vi "Format 2D Test Info Table.vi"(1 "Parameter Name Array":string[](array[string])) -> (0 "Parameter Table":string[][](array[string]))   [LabVIEW 2010]
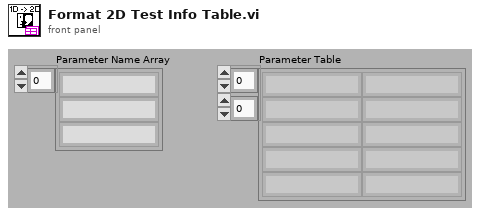
[diagram p1: front panel]
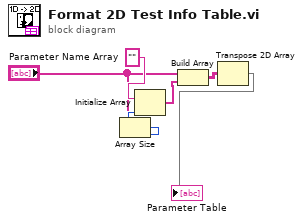
[diagram p0: block diagram]
diagram:
  n1 = Array Size(array="Parameter Name Array") -> (size(s)=w4:i32)
  n2 = Initialize Array("", w4) -> (w6:string[])
  n3 = Build Array("Parameter Name Array", w6) -> (w1:string[][])
  n4 = Transpose 2D Array(2D array=w1) -> (transposed array=→"Parameter Table":string[][])
